vi "Get Class Names.vi"(11 "Qualified names":string[](array[string])) -> (3 "Class names only":string[](array[string]))   [LabVIEW 2020, in "Report Generator.lvclass"]
uses:
  Report Generator.lvclass
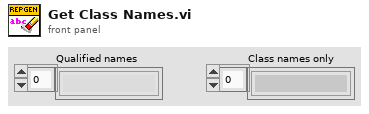
[diagram p1: front panel]
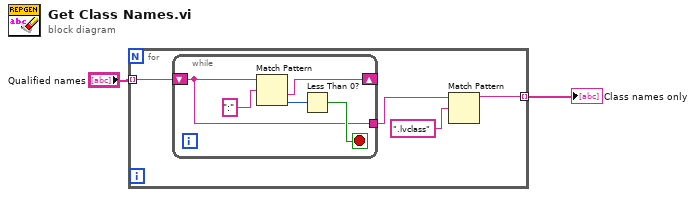
[diagram p0: block diagram]
diagram:
  n1 = for {
    tunnel: "Qualified names" -> [w6] mode=indexing
    tunnel: [w5] -> w1 mode=indexing
    n2 = while {
      shift-right: [w9] -> _
      shift-left: w6 -> [w7]
      tunnel: [w7] -> w3
      stop <- w8 stop-if-true
      n3 = Match Pattern(string=w7, regular expression=":") -> (after substring=w9:string, offset past match=w11:i32)  [unwired: 1 in, 2 out]
      n4 = Less Than 0?(x=w11) -> (x < 0?=w8:bool)
    }
    n5 = Match Pattern(string=w3, regular expression=".lvclass") -> (before substring=w5:string)  [unwired: 1 in, 3 out]
  }
  "Class names only" <- w1
